vi "Shared_DCPower_0V_Stop.vi"(9 "Settling Time (s)":dbl=0.01, 10 "Pins":tag[](array[tag]), 11 "Semiconductor Module Context":T1) -> (0 "error Out":errorcluster)   [LabVIEW 2023, in "Shared.lvlib"]
doc: "Set the Voltage Level to 0V and then stops supplying from System Power Supply for Relay control"
uses:
  Shared.lvlib
  <vilib>/NI_TestStand_SemiconductorModule/NI_TestStand_Semiconductor_Module.lvlibp/PinMap/General/SemiconductorModuleContext.ctl
  <vilib>/NI_TestStand_SemiconductorModule/NI_TestStand_Semiconductor_Module.lvlibp/PinMap/DC Power/PinsToNIDCPowerSessions.vi
  <vilib>/NI_TestStand_SemiconductorModule/NI_TestStand_Semiconductor_Module.lvlibp
  ResourceHandling/ResourceHandling.lvlib
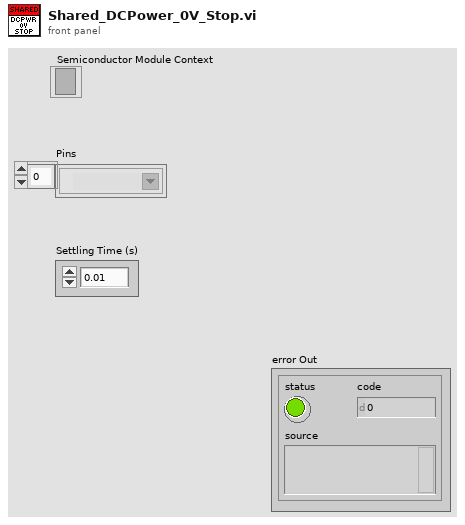
[diagram p1: front panel]
types:
  T1 = typedef "NI_TestStand_Semiconductor_Module.lvlibp/SemiconductorModuleContext.ctl" = refnum<k7>
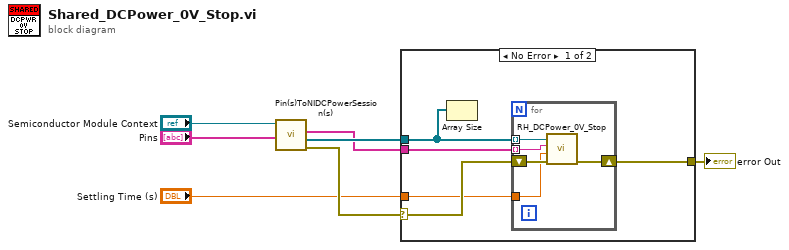
[diagram p0: block diagram]
diagram:
  n1 = call-poly <vilib>:"Pin(s)ToNIDCPowerSession(s).vi"("Pins"="Pins", "Semiconductor Module Context"="Semiconductor Module Context") -> ("error out"=w6:errorcluster, "Instrument Sessions"=w5:refnum<k15>[], "Channel Strings"=w4:string[])  [unwired: 5 in, 2 out]
  n2 = case shown="No Error" w6 {
    selector: w6 -> [w9 w18]
    tunnel: w5 -> [w12 _]
    tunnel: w4 -> [w11 _]
    tunnel: [w10 w18] -> w3
    tunnel: "Settling Time (s)" -> [w8 _]
    frame No Error {
      n3 = Array Size(array=w12) -> ()  [unwired: 1 out]
      n4 = for {
        tunnel: w12 -> [w17] mode=indexing
        tunnel: w11 -> [w16] mode=indexing
        shift-right: [w15] -> w10
        shift-left: w9 -> [w14]
        tunnel: w8 -> [w13]
        n5 = call "RH_DCPower_0V_Stop.vi"("error in (no error)"=w14, "Settling (s)"=w13, "Channel List"=w16, "DCPower Session In"=w17) -> ("error out"=w15:errorcluster)  [unwired: 6 in, 1 out]
      }
    }
    frame Error {
    }
  }
  "error Out" <- w3
